vi "Read args.vi"(8 "error in":errorcluster, 11 "Shared Library Module configuration in":refnum<class "Shared Library Module configuration.lvclass">) -> (0 "error out":errorcluster, 2 "args":string[](array[string]), 3 "Shared Library Module configuration out":refnum<class "Shared Library Module configuration.lvclass">)   [LabVIEW 2013, in "Shared Library Module configuration.lvclass"]
uses:
  Shared Library Module configuration.lvclass
  Shared Library Module configuration.lvclass/Shared Library Module configuration.ctl
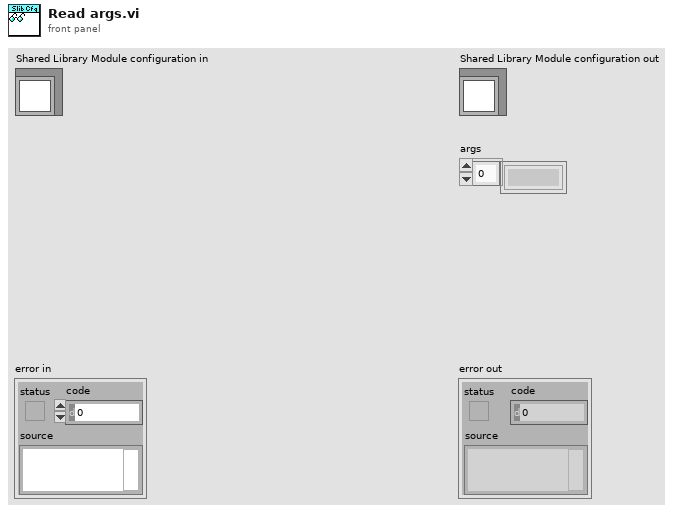
[diagram p1: front panel]
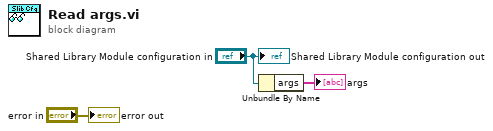
[diagram p0: block diagram]
diagram:
  n1 = Unbundle By Name("Shared Library Module configuration in") -> ("args"=→"args":string[])
  "error out" <- "error in"
  "Shared Library Module configuration out" <- "Shared Library Module configuration in"
